vi "Create Simulation Section.vi"(8 "error in (no error)":errorcluster, 11 "Parent Ref in":T1 format="%.0x") -> (0 "error out":errorcluster, 2 "Section Ptr":T1 format="%.0x", 3 "Parent Ref out":T1 format="%.0x")   [LabVIEW 2015, in "J1939 Addon Shared.lvlib"]
uses:
  J1939 Addon Shared.lvlib
  <vilib>/NI Veristand/Custom Device API/Custom Device Item Ref.ctl
  Constants.vi
  <vilib>/NI/NI VeriStand Advanced SysDef API/SysDef API/Advanced System Definition.lvlib
  <vilib>/NI VeriStand/Custom Device API/Custom Device API.lvlib
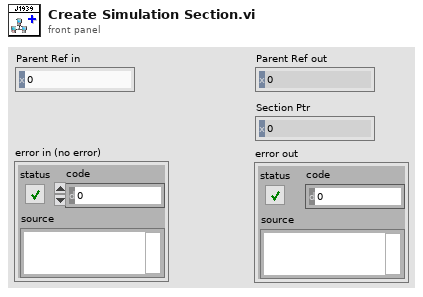
[diagram p1: front panel]
types:
  T1 = typedef "Custom Device API.lvlib/Custom Device Item Ref.ctl" = u64
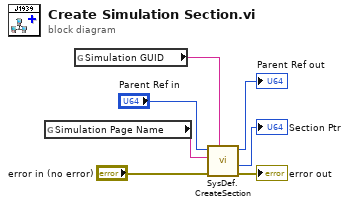
[diagram p0: block diagram]
diagram:
  n1 = global read "Constants.vi" "Simulation Page Name"() -> (w2:string)
  n2 = global read "Constants.vi" "Simulation GUID"() -> (w3:string)
  n3 = call <vilib>:"SysDef.CreateSection.vi"("GUID"=w3, "error in (no error)"="error in (no error)", "Name"=w2, "nodeID"="Parent Ref in") -> ("error out"=→"error out":errorcluster, "New NodeID"=→"Section Ptr":u64, "nodeID out"=→"Parent Ref out":u64)  [unwired: 4 in, 1 out]
